vi "sendAndWaitForResponse.vi"(8 "error in":errorcluster, 10 "Command":string="Test", 11 "NetworkConnection in":refnum<class "NetworkConnection.lvclass">) -> (0 "error out":errorcluster, 2 "Msg Id":i32, 3 "NetworkConnection out":refnum<class "NetworkConnection.lvclass">)   [LabVIEW 2020]
doc: "Provides a basic example of an RT user interface that uses network streams to connect to a PC.JKI Network Streams Connection 1.1.1.15\nJavier Ruiz - JKI\nCopyright (c) 2020, JKI\n\nThis library is provided \"AS IS\" ,WITHOUT WARRANTIES OR CONDITIONS OF ANY KIND, either express or implied."
uses:
  <vilib>/addons/_JKI.lib/Network_Streams_Connection.llb/NetworkConnection.lvclass
  <vilib>/addons/_JKI.lib/Network_Streams_Connection.llb/PublicSettings.ctl
  <vilib>/addons/_JKI.lib/Network_Streams_Connection.llb/NetworkCommand--Cluster.ctl
  <vilib>/addons/_JKI.lib/Network_Streams_Connection.llb/NetworkConnection.lvclass/NetworkConnection.ctl
  <userlib>/_MGI/Timing/MGI Wait/MGI Wait (U32).vi
panel:
  in  "Settings":T1
  out "Numeric":i32
  out "Connected?":bool
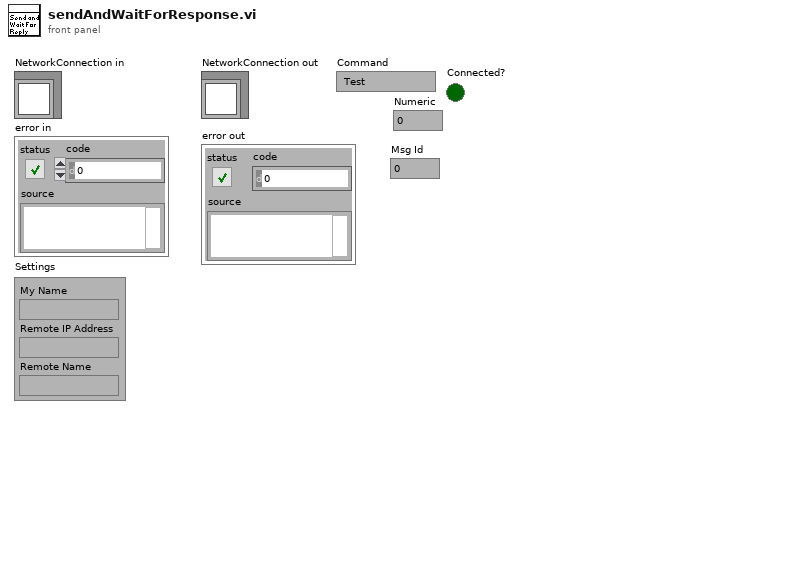
[diagram p1: front panel]
types:
  T1 = typedef "NetworkConnection.lvclass/PublicSettings.ctl" = cluster{"My Name":string, "Remote IP Address":string, "Remote Name":string}
  T2 = typedef "NetworkConnection.lvclass/NetworkCommand--Cluster.ctl" = cluster{"Command":string, "Arguments":variant, " Msg Id":i32}
  T3 = cluster{"Messages[0]":T2, "Messages[1]":T2, "Messages[2]":T2, "Messages[3]":T2, "Messages[4]":T2, "Messages[5]":T2, "Messages[6]":T2, "Messages[7]":T2, "Messages[8]":T2}
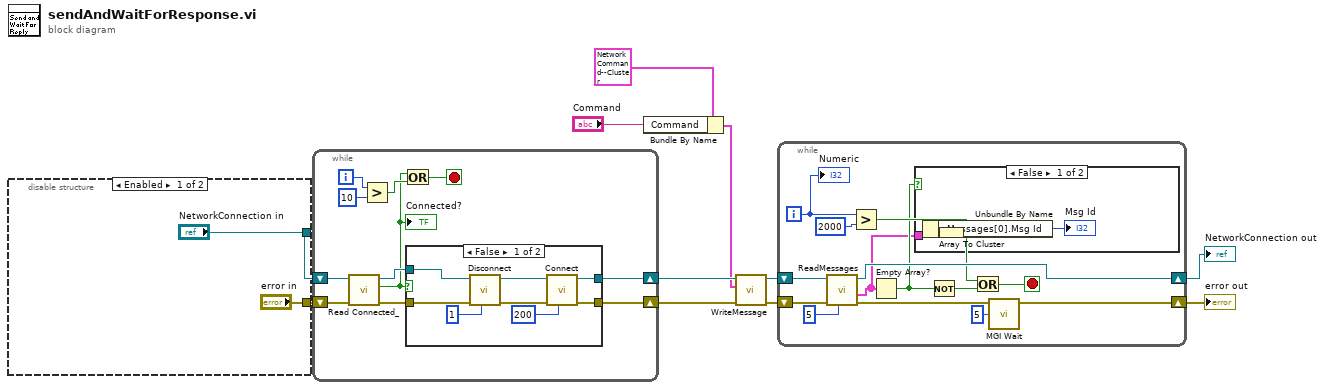
[diagram p0: block diagram]
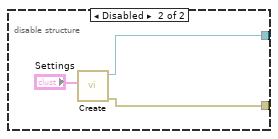
[diagram p2: hidden frame]
diagram:
  n1 = disable-structure shown="Enabled" {
    disable-tunnel: ["NetworkConnection in" w16] -> w2
    disable-tunnel: ["error in" w15] -> w1
    frame Enabled {
    }
    frame Disabled {
      n2 = call <vilib>:"Create.vi"("Settings"="Settings") -> ("error out"=w15:errorcluster, "NetworkConnection out"=w16:refnum<class "NetworkConnection.lvclass">)  [unwired: 9 in]
    }
  }
  n3 = while {
    shift-right: [w23] -> w10
    shift-left: w2 -> [w27]
    shift-right: [w22] -> w11
    shift-left: w1 -> [w26]
    i -> [w21]
    stop <- w18 stop-if-true
    n4 = call <vilib>:"Read Connected_.vi"("error in (no error)"=w26, "NetworkConnection in"=w27) -> ("error out"=w25:errorcluster, "Connected?"=w17:bool, "NetworkConnection out"=w24:refnum<class "NetworkConnection.lvclass">)  [unwired: 7 in]
    "Connected?" <- w17
    n5 = Greater?(x=w21, y=10) -> (0:w19:bool)
    n6 = Or(x=w17, y=w19) -> (x .or. y?=w18:bool)
    n7 = case shown="False" w17 {
      tunnel: w25 -> [w31 w36]
      tunnel: w24 -> [w33 w37]
      tunnel: [w34 w37] -> w23
      tunnel: [w35 w36] -> w22
      frame False {
        n8 = call <vilib>:"Disconnect.vi"("Timeout ms (1000)"=1 ("(ms)"), "error in (no error)"=w31, "NetworkConnection in"=w33) -> ("error out"=w30:errorcluster, "NetworkConnection out"=w32:refnum<class "NetworkConnection.lvclass">)  [unwired: 7 in]
        n9 = call <vilib>:"Connect.vi"("Timeout(ms)"=200, "error in (no error)"=w30, "NetworkConnection in"=w32) -> ("error out"=w35:errorcluster, "NetworkConnection out"=w34:refnum<class "NetworkConnection.lvclass">)  [unwired: 6 in, 1 out]
      }
      frame True {
      }
    }
  }
  n10 = Bundle By Name(cluster=T2 {"Command"="", "Arguments"=variant, " Msg Id"=0} ("Message"), "Command"="Command") -> (w4:T2)
  n11 = call <vilib>:"WriteMessage.vi"("error in (no error)"=w11, "Message"=w4, "NetworkConnection in"=w10) -> ("error out"=w8:errorcluster, "NetworkConnection out"=w9:refnum<class "NetworkConnection.lvclass">)  [unwired: 5 in, 2 out]
  n12 = while {
    shift-right: [w51] -> w7
    shift-left: w9 -> [w49]
    shift-right: [w42] -> w6
    shift-left: w8 -> [w48]
    i -> [w47]
    stop <- w50 stop-if-true
    n13 = call <vilib>:"ReadMessages.vi"("Timeout(ms)"=5, "error in (no error)"=w48, "NetworkConnection in"=w49) -> ("error out"=w43:errorcluster, "Messages"=w38:T2[], "NetworkConnection out"=w51:refnum<class "NetworkConnection.lvclass">)  [unwired: 4 in, 2 out]
    n14 = Greater?(x=w47, y=2000) -> (0:w45:bool)
    n15 = Empty Array?(array=w38) -> (empty?=w39:bool)
    n16 = case shown="False" w39 {
      tunnel: w38 -> [w54 _]
      frame False {
        n17 = Array To Cluster(array=w54) -> (cluster=w53:T3)
        n18 = Unbundle By Name(w53) -> ("Messages[0].Msg Id"=→"Msg Id":i32)
      }
      frame True {
      }
    }
    n19 = Not(x=w39) -> (.not. x?=w40:bool)
    n20 = Or(x=w45, y=w40) -> (x .or. y?=w50:bool)
    n21 = call-poly <userlib>:"MGI Wait.vi"("ms"=u32 5, "Error In"=w43) -> ("Error Out"=w42:errorcluster)  [unwired: 5 in]
    "Numeric" <- w47
  }
  "NetworkConnection out" <- w7
  "error out" <- w6
